vi "Configure Delete Panel_Msg.vi"(8 "error in (no error)":errorcluster, 10 "Ctl Ref":refnum<vi>, 11 "Delete Panel Control_Msg":refnum<class "Delete Control_Behavior.lvclass">) -> (0 "error out":errorcluster, 3 "Delete Panel Control_Msg":refnum<class "Delete Control_Behavior.lvclass">)   [LabVIEW 2015, in "Delete Control_Behavior.lvclass"]
doc: "This VI sends the message to an actor."
uses:
  Delete Control_Behavior.lvclass
  Delete Control_Behavior.lvclass/Delete Control_Behavior.ctl
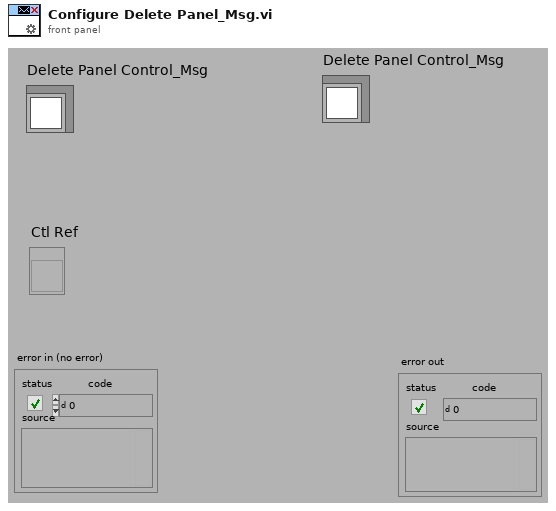
[diagram p1: front panel]
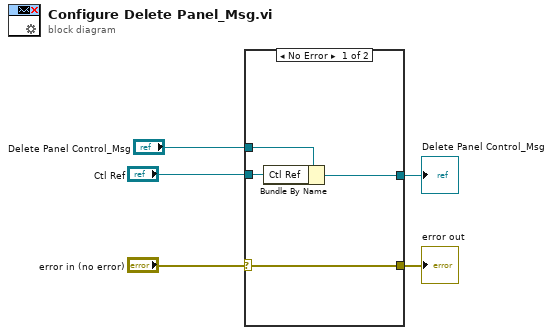
[diagram p0: block diagram]
diagram:
  n1 = case shown="No Error" "error in (no error)" {
    selector: "error in (no error)" -> [w6 w11]
    tunnel: "Delete Panel Control_Msg" -> [w9 w10]
    tunnel: "Ctl Ref" -> [w8 _]
    tunnel: [w7 w10] -> w3
    tunnel: [w6 w11] -> w1
    frame No Error {
      n2 = Bundle By Name(cluster=w9, "Ctl Ref"=w8) -> (w7:refnum<class "Delete Control_Behavior.lvclass">)
    }
    frame Error {
    }
  }
  "error out" <- w1
  "Delete Panel Control_Msg" <- w3
